vi "PPMS.GET ALL.vi"(8 "error in (no error)":errorcluster, 11 "instrument.PPMS":refnum<class "instrument.PPMS.lvclass">) -> (0 "error out":errorcluster, 2 "getAll":T1, 3 "instrument.PPMS out":refnum<class "instrument.PPMS.lvclass">)   [LabVIEW 2019, in "instrument.PPMS.lvclass"]
uses:
  instrument.PPMS.lvclass
  Typedefs/PPMS.getAll--cluster.ctl
  51190d81-5331-44c5-ae51-655eeb647297.vi
  51190d81-5331-44c5-ae51-655eeb647297.vi/80ce59d7-09bc-4796-af77-66e66d4f99ec.vi
  51190d81-5331-44c5-ae51-655eeb647297.vi/91fffe2f-4afc-4961-a6cf-a70d969ed2f8.vi
  51190d81-5331-44c5-ae51-655eeb647297.vi/80ce59d7-09bc-4796-af77-66e66d4f99ec.vi/e34b2247-da76-4b56-a3f4-ce5512ab0c2f.vi
  51190d81-5331-44c5-ae51-655eeb647297.vi/80ce59d7-09bc-4796-af77-66e66d4f99ec.vi/454e9f09-60ee-47dc-b65c-c59ab56f1143.vi
  51190d81-5331-44c5-ae51-655eeb647297.vi/91fffe2f-4afc-4961-a6cf-a70d969ed2f8.vi/6ea83089-af52-4f98-9799-be36018295d6.vi
  51190d81-5331-44c5-ae51-655eeb647297.vi/80ce59d7-09bc-4796-af77-66e66d4f99ec.vi/454e9f09-60ee-47dc-b65c-c59ab56f1143.vi/86746460-9620-49d8-8502-15c297c54def.vi
  <userlib>/LevyLab/Levylab Instruments/SMOs/RemoteControl/API/Remote Client.vi
  <vilib>/JDP Science/JSONtext/JSON text to Variant.vi
  <vilib>/JDP Science/JSONtext/LVClass Serializer/JSONtext LVClass Serializer.lvclass
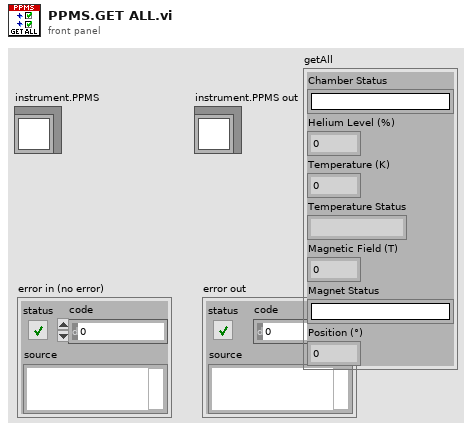
[diagram p1: front panel]
types:
  T1 = typedef "instrument.PPMS.lvclass/PPMS.getAll--cluster.ctl" = cluster{"Chamber Status":string, "Helium Level (%)":dbl, "Temperature (K)":dbl, "Temperature Status":string, "Magnetic Field (T)":dbl, "Magnet Status":string, "Position (°)":dbl}
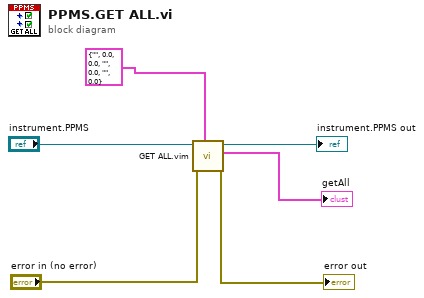
[diagram p0: block diagram]
diagram:
  n1 = call "GET ALL.vim"("type"=T1 {"Chamber Status"="", "Helium Level (%)"=0.0, "Temperature (K)"=0.0, "Temperature Status"="", "Magnetic Field (T)"=0.0, "Magnet Status"="", "Position (°)"=0.0} ("getAll"), "error in (no error)"="error in (no error)", "Instrument in"="instrument.PPMS") -> ("error out"=→"error out":errorcluster, "getAll"=→"getAll":T1, "Instrument out"=→"instrument.PPMS out":refnum<class "instrument.PPMS.lvclass">)  [unwired: 6 in]
